vi "Create Task.vi"(6 "Authorization":T1[](array[typedef]), 8 "error in (no error)":errorcluster, 9 "Description":string, 10 "Name":string, 11 "Project GID":string) -> (0 "error out":errorcluster, 2 "gid":string)   [LabVIEW 2016]
uses:
  <vilib>/addons/_JKI.lib/REST Client/classes/REST Client/HTTP Header.ctl
  <vilib>/addons/_JKI.lib/REST Client/classes/REST Client/REST Client.lvclass
  <vilib>/addons/_JKI.lib/Serialization/JSON/JKI JSON Serialization.lvlib
panel:
  out "Response body":string
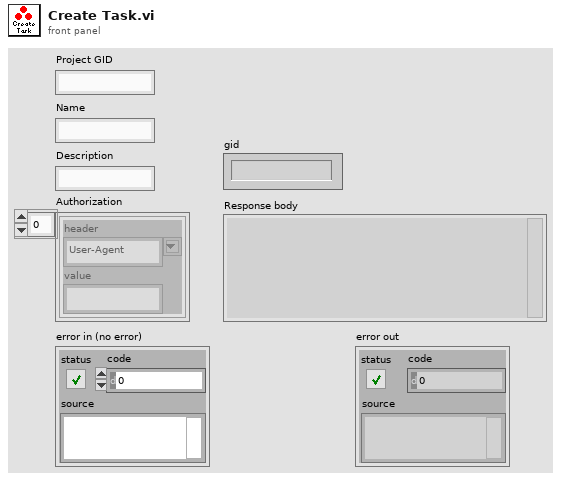
[diagram p1: front panel]
types:
  T1 = typedef "REST Client.lvlib/REST Client.lvclass/HTTP Header.ctl" = cluster{"header":string, "value":string}
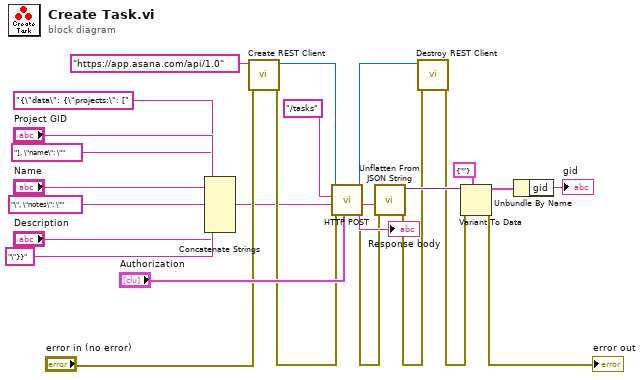
[diagram p0: block diagram]
diagram:
  n1 = Concatenate Strings("{\"data\": {\"projects:\": [", "Project GID", "], \"name\": \"" ("string"), "Name", "\", \"notes\": \"" ("string"), "Description", "\"}}" ("string")) -> (w15:string)
  n2 = call <vilib>:"Create REST Client.vi"("error in (no error)"="error in (no error)", "Base URL"="https://app.asana.com/api/1.0") -> ("error out"=w18:errorcluster, "REST Client out"=w22:refnum<class "REST Client.lvclass">)  [unwired: 8 in]
  n3 = call-dynamic "HTTP POST.vi"("request specific headers"="Authorization", "error in (no error)"=w18, "Request body"=w15, "Path"="/tasks", "REST Client in"=w22) -> ("error out"=w12:errorcluster, "Response body"=w13:string, "REST Client out"=w21:refnum<class "REST Client.lvclass">)  [unwired: 1 in, 3 out]
  "Response body" <- w13
  n4 = call <vilib>:"Unflatten From JSON String.vi"("error in (no error)"=w12, "JSON String"=w13) -> ("error out"=w11:errorcluster, "Variant"=w14:variant)  [unwired: 8 in]
  n5 = call-dynamic "Destroy REST Client.vi"("error in (no error)"=w11, "REST Client in"=w21) -> ("error out"=w10:errorcluster)  [unwired: 9 in]
  n6 = Variant To Data(error in=w10, type=cluster{"gid":string} {"gid"=""}, Variant=w14) -> (data=w7:cluster{"gid":string}, error out=→"error out":errorcluster)
  n7 = Unbundle By Name(w7) -> ("gid"=→"gid":string)
